vi "WPI_CAN_PCMReceive.vi"(11 "Pneumatics Control Module (0)":u8) -> (3 "Pneumatics Control Module Out":u8)   [LabVIEW 2017]
uses:
  <vilib>/Rock Robotics/WPI/CAN/PCM/WPI_CAN_PCMMessageIDs.ctl
  <vilib>/Rock Robotics/WPI/CAN/PCM/WPI_CAN_PCMGlobalOps.ctl
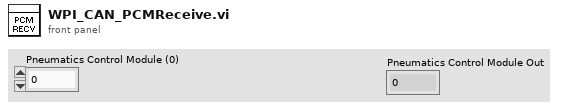
[diagram p1: front panel]
types:
  T1 = cluster{"Solenoid Status":bool[], "Battery Voltage":dbl, "Solenoid Voltage":dbl, "Compressor Current":dbl, "Status":cluster{"CompressorEnabled":bool, "StickySolenoidFault":bool, "StickyCompressorFault":bool, "SolenoidFault":bool, "CompressorFault":bool, "HardwareFault":bool, "ClosedLoopStatus":bool, "PressureStatus":bool}, "Module Enabled":bool, "ClosedLoopSuggestedOutput":bool, "CAN Error":errorcluster, "Sticky Solenoid Faults":bool[]}
  T2 = typedef "WPI_CAN_PCMMessageIDs.ctl" = u32
  T3 = typedef "WPI_CAN_PCMGlobalOps.ctl" = enum16{"Read For Send", "Write After Receive", "Set Solenoids", "Set Closed Loop", "Clear Sticky Faults", "Get All", "Write Error", "Write After Receive Blacklist", "Set Control Frame Rate"}
  T4 = cluster{"Boolean array[0]":bool, "Boolean array[1]":bool, "Boolean array[2]":bool, "Boolean array[3]":bool, "Boolean array[4]":bool, "Boolean array[5]":bool, "Boolean array[6]":bool, "Boolean array[7]":bool}
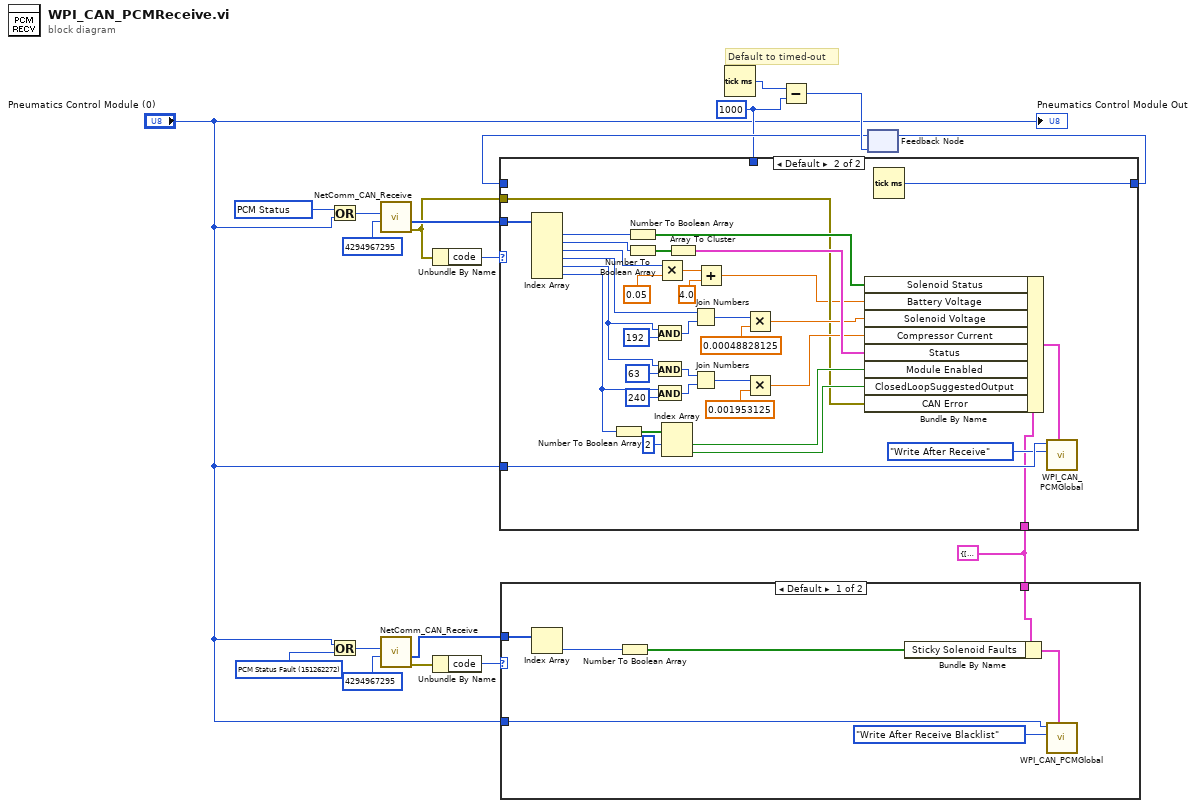
[diagram p0: block diagram]
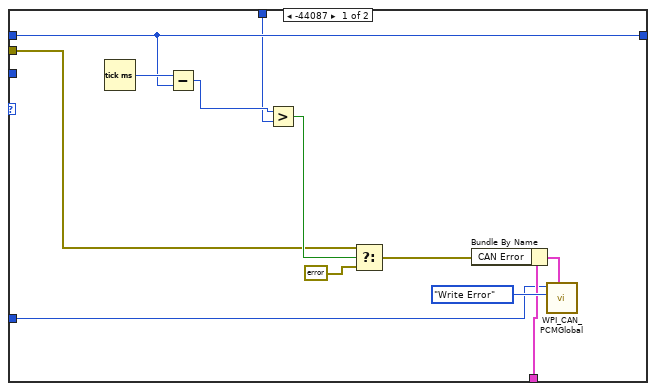
[diagram p3: hidden frame]
diagram:
  w2 = u32 1000 ("y")
  w7 = T1 {"Solenoid Status"=[], "Battery Voltage"=0.0, "Solenoid Voltage"=0.0, "Compressor Current"=0.0, "Status"={"CompressorEnabled"=FALSE, "StickySolenoidFault"=FALSE, "StickyCompressorFault"=FALSE, "SolenoidFault"=FALSE, "CompressorFault"=FALSE, "HardwareFault"=FALSE, "ClosedLoopStatus"=FALSE, "PressureStatus"=FALSE}, "Module Enabled"=FALSE, "ClosedLoopSuggestedOutput"=FALSE, "CAN Error"={"status"=FALSE, "code"=0, "source"=""}, "Sticky Solenoid Faults"=[]} ("Write After Receive")
  w12 = T2 151262272 items=["PCM Control"=151264256, "PCM Status"=151262208, "PCM Status Fault"=151262272, "PCM Debug"=151262336]
  w17 = T2 151262208 items=["PCM Control"=151264256, "PCM Status"=151262208, "PCM Status Fault"=151262272, "PCM Debug"=151262336]
  # "Default to timed-out"
  n1 = Or(x=w17, y="Pneumatics Control Module (0)") -> (x .or. y?=w18:T2)
  n2 = Or(x="Pneumatics Control Module (0)", y=w12) -> (x .or. y?=w11:T2)
  n3 = call <vilib>:"NetComm_CAN_Receive.vi"("Message ID Mask"=u32 4294967295, "Message ID"=w18) -> ("error out"=w15:errorcluster, "Data"=w19:u8[])  [unwired: 6 in, 2 out]
  n4 = call <vilib>:"NetComm_CAN_Receive.vi"("Message ID Mask"=u32 4294967295, "Message ID"=w11) -> ("error out"=w10:errorcluster, "Data"=w8:u8[])  [unwired: 6 in, 2 out]
  n5 = Unbundle By Name(w15) -> ("code"=w14:i32)
  n6 = Unbundle By Name(w10) -> ("code"=w9:i32)
  n7 = case shown="Default" w9 {
    tunnel: w8 -> [w26 _]
    tunnel: "Pneumatics Control Module (0)" -> [w23 _]
    tunnel: w7 -> [w22 _]
    frame Default {
      n8 = Index Array(array=w26) -> (element=w25:u8)  [unwired: 1 in]
      n9 = Number To Boolean Array(number=w25) -> (Boolean array=w21:bool[])
      n10 = Bundle By Name(cluster=w22, "Sticky Solenoid Faults"=w21) -> (w20:T1)
      n11 = call <vilib>:"WPI_CAN_PCMGlobal.vi"("Write After Receive"=w20, "Operation"=WPI_CAN_PCMGlobalOps."Write After Receive Blacklist", "Pneumatics Control Module (0)"=w23) -> ()  [unwired: 6 in, 3 out]
    }
    frame -44087 {
    }
  }
  n12 = Tick Count (ms)() -> (millisecond timer value=w5:u32)
  n13 = Subtract(x=w5, y=w2) -> (x-y=w6:u32)
  n14 = feedback #1(w6) -> (w3:u32)
  n15 = case shown="Default" w14 {
    tunnel: "Pneumatics Control Module (0)" -> [w27 w74]
    tunnel: w19 -> [_ w73]
    tunnel: w15 -> [w32 w43]
    tunnel: w7 -> [w30 w42]
    tunnel: [w34 w39] -> w4
    tunnel: w3 -> [w34 _]
    tunnel: w2 -> [w33 _]
    frame -44087 {
      n16 = Tick Count (ms)() -> (millisecond timer value=w38:u32)
      n17 = Subtract(x=w38, y=w34) -> (x-y=w37:u32)
      n18 = Greater?(x=w37, y=w33) -> (0:w36:bool)
      n19 = Select(t=w32, s=w36, f=errorcluster {"status"=FALSE, "code"=0, "source"=""}) -> (s? t:f=w28:errorcluster)
      n20 = Bundle By Name(cluster=w30, "CAN Error"=w28) -> (w29:T1)
      n21 = call <vilib>:"WPI_CAN_PCMGlobal.vi"("Write After Receive"=w29, "Operation"=WPI_CAN_PCMGlobalOps."Write Error", "Pneumatics Control Module (0)"=w27) -> ()  [unwired: 6 in, 3 out]
    }
    frame Default {
      n22 = Index Array(array=w73) -> (element #1=w72:u8, element #2=w71:u8, element #3=w69:u8, element #4=w67:u8, element #5=w54:u8, element #6=w56:u8)  [unwired: 6 in]
      n23 = Number To Boolean Array(number=w56) -> (Boolean array=w60:bool[])
      n24 = Number To Boolean Array(number=w72) -> (Boolean array=w50:bool[])
      n25 = Number To Boolean Array(number=w71) -> (Boolean array=w70:bool[])
      n26 = And(x=w54, y=u8 192) -> (x .and. y?=w53:u8)
      n27 = And(x=w54, y=u8 63) -> (x .and. y?=w61:u8)
      n28 = And(x=w56, y=u8 240) -> (x .and. y?=w57:u8)
      n29 = Multiply(x=w69, y=0.05) -> (x*y=w46:dbl)
      n30 = Index Array(array=w60, index #1=2 ("index")) -> (element #1=w45:bool, element #2=w44:bool)  [unwired: 1 in]
      n31 = Array To Cluster(array=w70) -> (cluster=w49:T4)
      n32 = Join Numbers(hi=w67, lo=w53) -> ((hi.lo)=w65:u16)
      n33 = Join Numbers(hi=w61, lo=w57) -> ((hi.lo)=w63:u16)
      n34 = Add(x=w46, y=4.0 ("x")) -> (x+y=w41:dbl)
      n35 = Multiply(x=w65, y=0.00048828125) -> (x*y=w48:dbl)
      n36 = Multiply(x=w63, y=0.001953125) -> (x*y=w47:dbl)
      n37 = Bundle By Name(cluster=w42, "Solenoid Status"=w50, "Battery Voltage"=w41, "Solenoid Voltage"=w48, "Compressor Current"=w47, "Status"=w49, "Module Enabled"=w45, "ClosedLoopSuggestedOutput"=w44, "CAN Error"=w43) -> (w51:T1)
      n38 = Tick Count (ms)() -> (millisecond timer value=w39:u32)
      n39 = call <vilib>:"WPI_CAN_PCMGlobal.vi"("Write After Receive"=w51, "Operation"=WPI_CAN_PCMGlobalOps."Write After Receive", "Pneumatics Control Module (0)"=w74) -> ()  [unwired: 6 in, 3 out]
    }
  }
  n40 = feedback-in #1(w4) -> ()
  "Pneumatics Control Module Out" <- "Pneumatics Control Module (0)"
